vi "FPGAPowerMeasurementAverage.vi"() -> ()   [LabVIEW 2009]
panel:
  out "Current":dynamicdata(graph)
  out "Voltage at FPGA":dynamicdata(graph)
  out "Power Signal":dynamicdata(graph)
  out "Average Voltage":dbl
  out "Average Current":dbl
  out "Average Power":dbl
  out "Voltages":dynamicdata(graph)
  in  "Number of Waveforms to Average":i32
  in  "rate":dbl=2000000.0
  in  "number of samples":i32=2000000
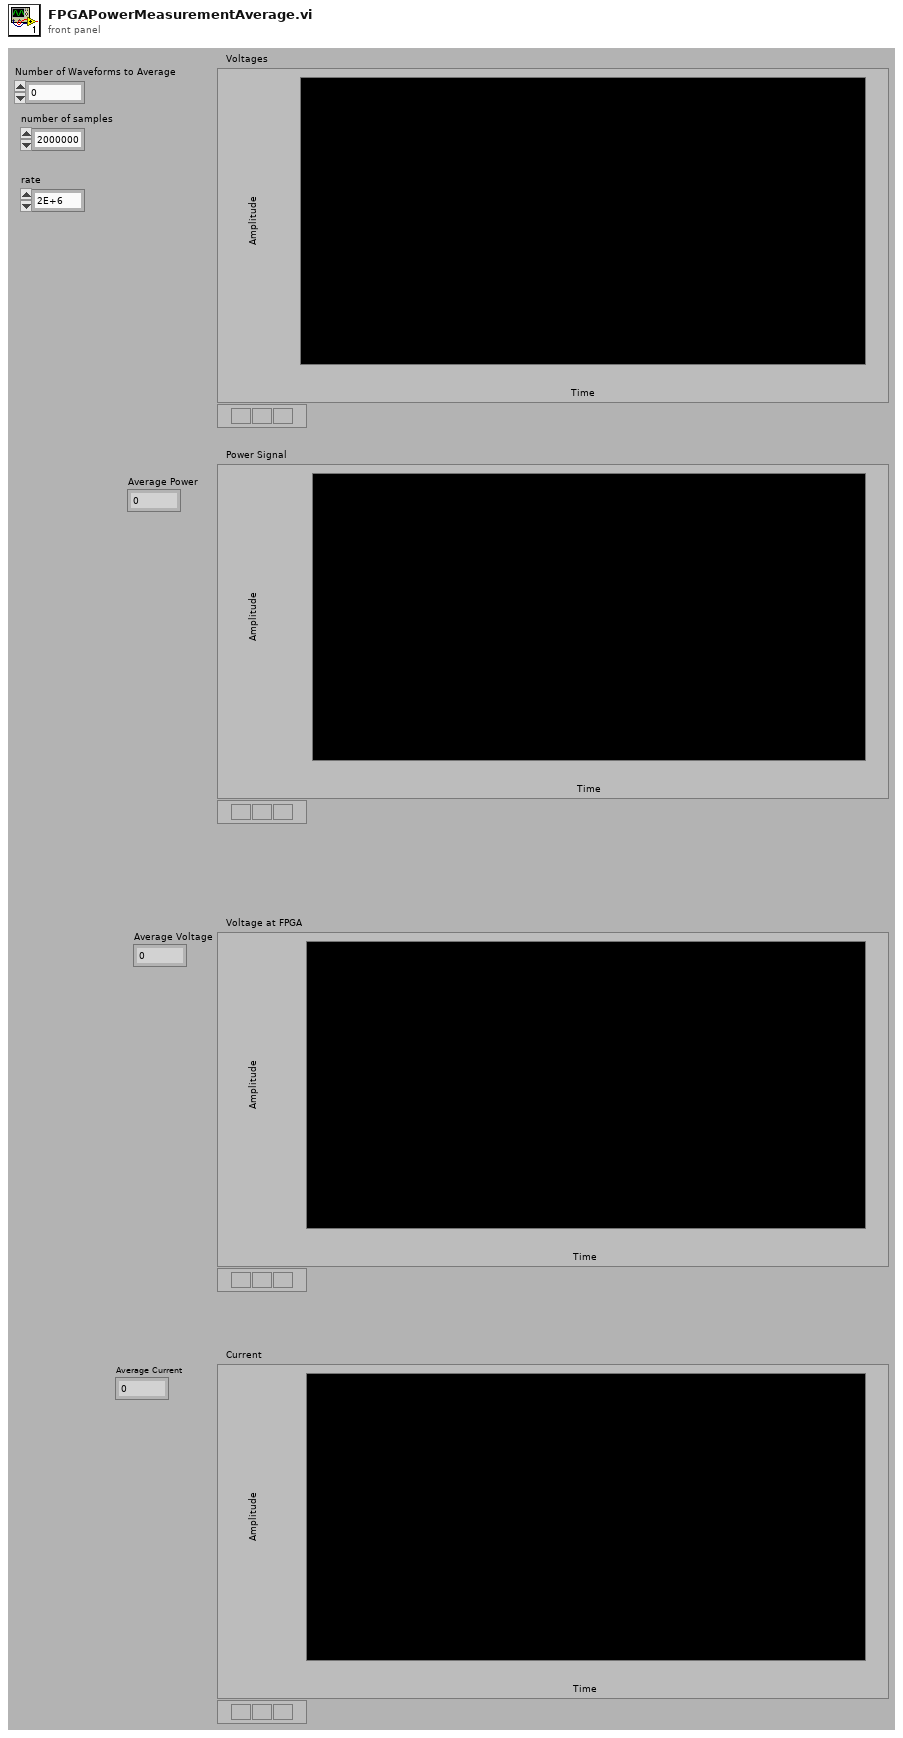
[diagram p1: front panel]
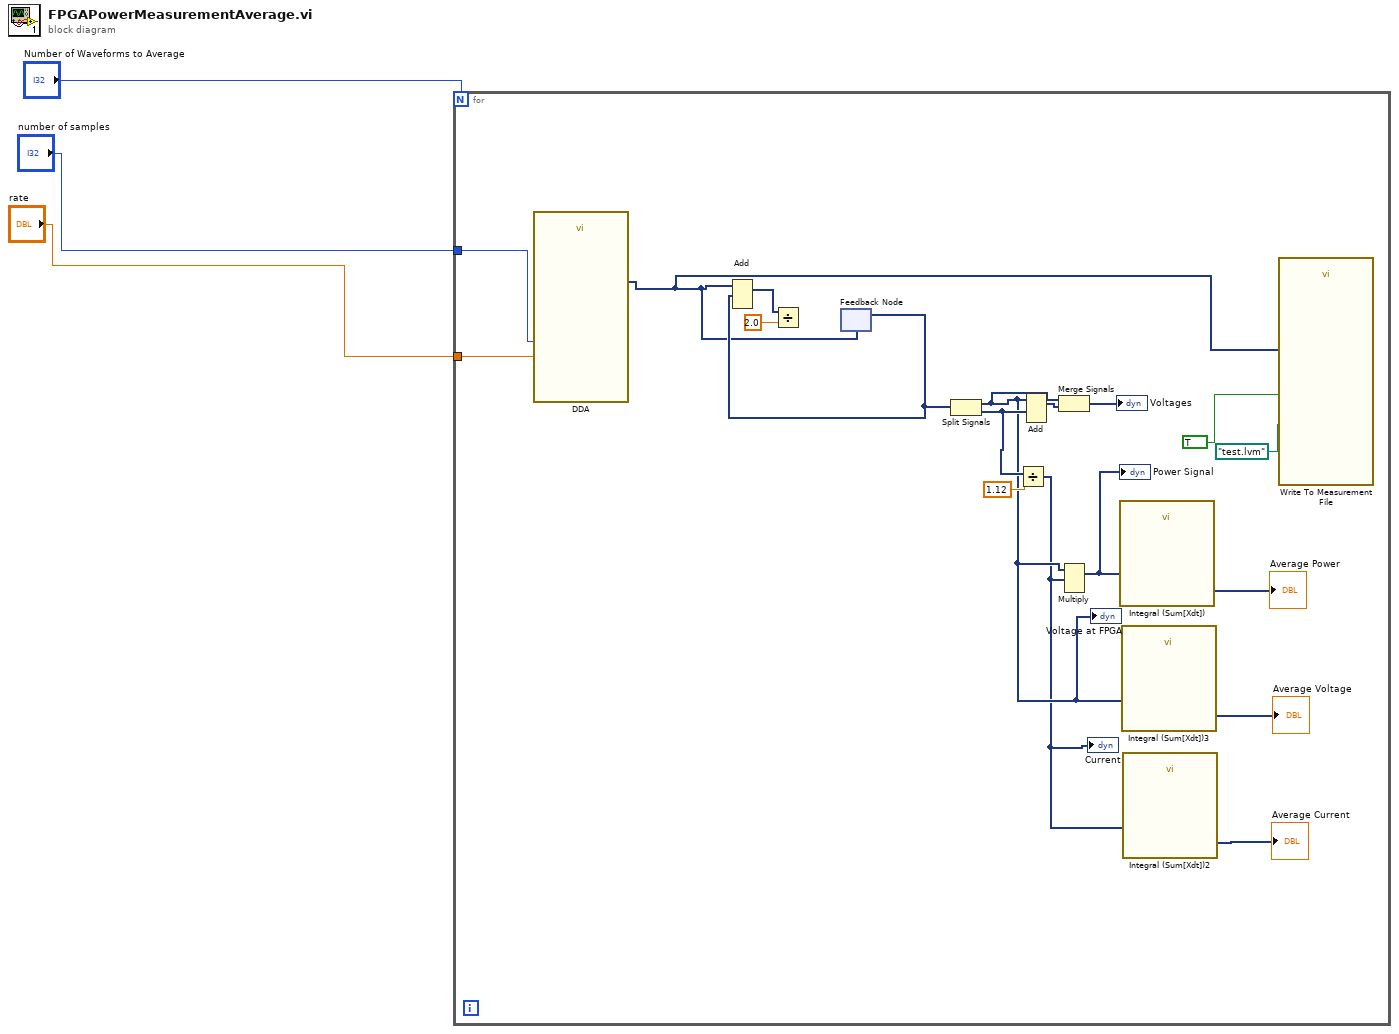
[diagram p0: block diagram]
diagram:
  n1 = for {
    N: "Number of Waveforms to Average" -> [_]
    tunnel: "number of samples" -> [w16]
    tunnel: "rate" -> [w15]
    n2 = call "DDA.vi"("rate"=w15, "number of samples"=w16) -> ("data"=w4:dynamicdata)  [unwired: 15 in, 2 out]
    n3 = feedback #1(w4) -> (w18:dynamicdata)
    n4 = Add(1:w18, 2:w4) -> (0:w22:dynamicdata)  [unwired: 1 in, 1 out]
    n5 = Divide(x=w22, y=2.0) -> (x/y=w20:dynamicdata)
    n6 = Split Signals(w18) -> (w8:dynamicdata, w10:dynamicdata)  [unwired: 2 in]
    "Voltage at FPGA" <- w8
    n7 = Divide(x=w10, y=1.12) -> (x/y=w7:dynamicdata)
    "Current" <- w7
    n8 = Add(1:w10, 2:w8) -> (0:w19:dynamicdata)  [unwired: 1 in, 1 out]
    n9 = Merge Signals(w8, w19) -> (→"Voltages":dynamicdata)
    n10 = Multiply(1:w7, 2:w8) -> (0:w9:dynamicdata)  [unwired: 1 in, 1 out]
    "Power Signal" <- w9
    n11 = call "Integral (Sum[Xdt])"("Signals"=w9) -> ("Result"=→"Average Power":dynamicdata)  [unwired: 5 in, 1 out]
    n12 = call "Integral (Sum[Xdt])3"("Signals"=w8) -> ("Result"=→"Average Voltage":dynamicdata)  [unwired: 5 in, 1 out]
    n13 = call "Integral (Sum[Xdt])2"("Signals"=w7) -> ("Result"=→"Average Current":dynamicdata)  [unwired: 5 in, 1 out]
    n14 = call "Write To Measurement File"("Signals"=w4, "Enable"=TRUE, "Filename"=path "test.lvm") -> ()  [unwired: 14 in, 3 out]
  }
